vi "Remove Last Item from Peek Stack.vi"(8 "error in (no error)":errorcluster, 11 "Data Cluster in":T1) -> (0 "error out":errorcluster, 2 "Removed VI":string, 3 "Data Cluster out":T1)   [LabVIEW 2020, in "Peek Window.lvlib"]
uses:
  Peek Window.lvlib
  MHL Data Cluster.ctl
  Open Diagram Argument--cluster.ctl
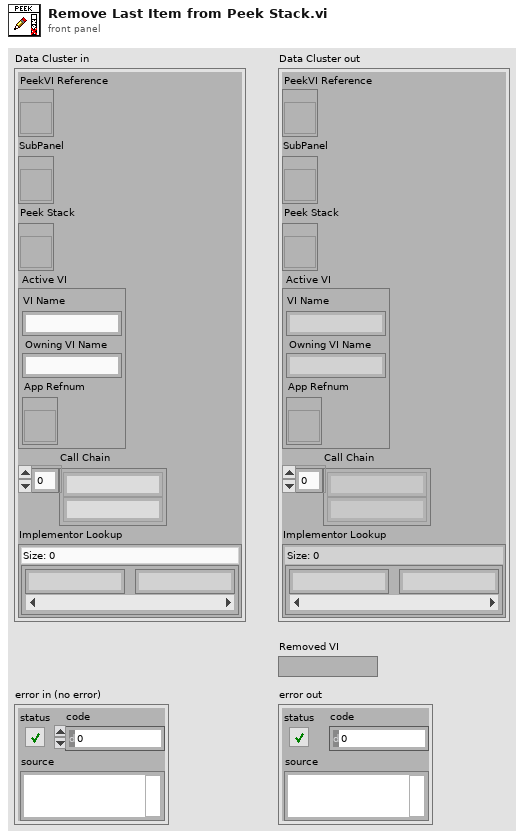
[diagram p1: front panel]
types:
  T1 = typedef "Peek Window.lvlib/MHL Data Cluster.ctl" = cluster{"PeekVI Reference":refnum<vi>, "SubPanel":refnum<vi>, "Peek Stack":refnum<vi>, "Active VI":T2, "Call Chain":string[], "Implementor Lookup":map{string, string}}
  T2 = typedef "Peek Window.lvlib/Open Diagram Argument--cluster.ctl" = cluster{"VI Name":string, "Owning VI Name":string, "App Refnum":refnum<vi>}
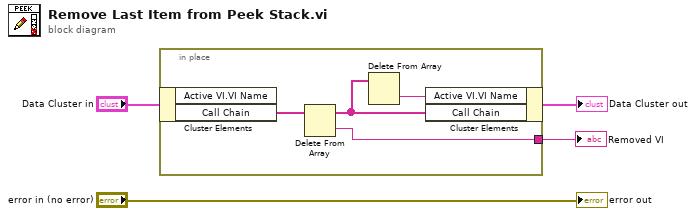
[diagram p0: block diagram]
diagram:
  n1 = in-place {
    in-place-border: [w7] -> w1
    n2 = in-place-cluster #1("Data Cluster in") -> ("Call Chain"=w8:string[])  [unwired: 1 out]
    n3 = Delete From Array(array=w8) -> (deleted portion=w7:string, array with subset deleted=w6:string[])  [unwired: 2 in]
    n4 = Delete From Array(array=w6) -> (deleted portion=w5:string)  [unwired: 2 in, 1 out]
    n5 = in-place-cluster #1("Active VI.VI Name"=w5, "Call Chain"=w6) -> (→"Data Cluster out":T1)
  }
  "Removed VI" <- w1
  "error out" <- "error in (no error)"
